vi "Launch Nested Analog Reader Actor.vi"(8 "error in (no error)":errorcluster, 10 "Nested Analog Reader Actor":refnum<class "Analog Reader.lvclass">, 11 "Caller Actor in":refnum<class "Actor.lvclass">) -> (0 "error out":errorcluster, 1 "Analog Input Current Values":refnum<queue>, 2 "Nested Actor's Enqueue":refnum<class "Message Enqueuer.lvclass">, 3 "Caller Actor out":refnum<class "Actor.lvclass">)   [LabVIEW 2024, in "DAQmx Actor.lvlib" / "Analog Reader.lvclass"]
uses:
  Analog Reader.lvclass
  <vilib>/ActorFramework/Actor/Actor.lvclass
  <vilib>/ActorFramework/Message Enqueuer/Message Enqueuer.lvclass
  Analog Reader.lvclass/Analog Reader.ctl
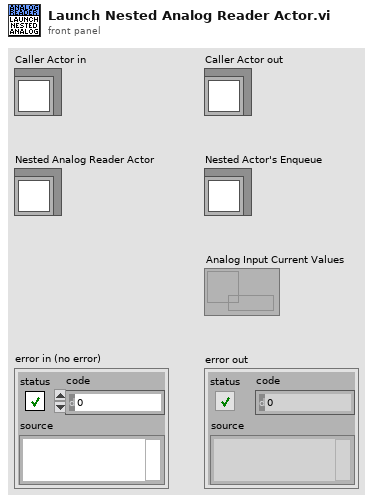
[diagram p1: front panel]
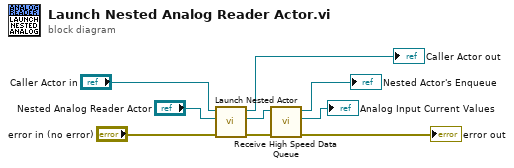
[diagram p0: block diagram]
diagram:
  n1 = call <vilib>:"Launch Nested Actor.vi"("error in (no error)"="error in (no error)", "Nested Actor"="Nested Analog Reader Actor", "Caller Actor in"="Caller Actor in") -> ("error out"=w5:errorcluster, "Nested Actor's Enqueuer"=w7:refnum<class "Message Enqueuer.lvclass">, "Caller Actor out"=→"Caller Actor out":refnum<class "Actor.lvclass">)  [unwired: 6 in]
  n2 = call "Receive High Speed Data Queue.vi"("error in (no error)"=w5, "Message Enqueuer"=w7) -> ("error out"=→"error out":errorcluster, "High Speed Data Queue"=→"Analog Input Current Values":refnum<queue>, "Message Enqueuer out"=→"Nested Actor's Enqueue":refnum<class "Message Enqueuer.lvclass">)  [unwired: 7 in]
